vi "1 File IO ex 10.vi"() -> ()   [LabVIEW 2015]
panel:
  in  "Stop":bool
  # "Temperature"
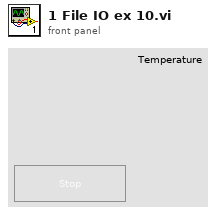
[diagram p1: front panel]
types:
  T1 = enum16{"open", "replace", "create", "open or create", "replace or create", "replace or create with confirmation"}
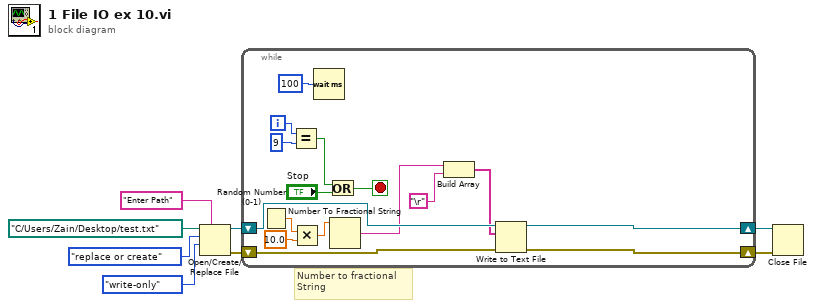
[diagram p0: block diagram]
diagram:
  # "Number to fractional \nString"
  n1 = Open/Create/Replace File(file path (use dialog)=path "C:/Users/Zain/Desktop/test.txt", prompt="Enter Path", operation (0:open)=T1."replace or create", access (0:read/write)=enum16{"read/write", "read-only", "write-only"}."write-only") -> (refnum out=w6:refnum<file>, error out=w5:errorcluster)  [unwired: 1 in, 2 out]
  n2 = while {
    shift-right: [w20] -> w4
    shift-left: w6 -> [w22]
    shift-right: [w19] -> w3
    shift-left: w5 -> [w21]
    i -> [w15]
    stop <- w23 stop-if-true
    n3 = Random Number (0-1)() -> (number: 0 to 1=w17:dbl)
    n4 = Equal?(x=w15, y=9) -> (x = y?=w13:bool)
    n5 = Multiply(x=w17, y=10.0) -> (x*y=w12:dbl)
    n6 = Wait (ms)(milliseconds to wait=u32 100) -> ()  [unwired: 1 out]
    n7 = Or(x=w13, y="Stop") -> (x .or. y?=w23:bool)
    n8 = Number To Fractional String(number=w12) -> (F-format string=w11:string)  [unwired: 3 in]
    n9 = Build Array(w11, "\r") -> (w9:string[])
    n10 = Write to Text File(file (use dialog)=w22, text=w9, error in=w21) -> (refnum out=w20:refnum<file>, error out=w19:errorcluster)  [unwired: 1 in, 1 out]
  }
  n11 = Close File(refnum=w4, error in=w3) -> ()  [unwired: 2 out]
